vi "Write Toggle enable.vi"(8 "error in (no error)":errorcluster, 10 "Toggle enable":bool, 11 "Motor-Maxon in":refnum<class "Motor-Maxon.lvclass">) -> (0 "error out":errorcluster, 3 "Motor-Maxon out":refnum<class "Motor-Maxon.lvclass">)   [LabVIEW 2013, in "PowderDeposition.lvlib" / "Motor-Maxon.lvclass"]
uses:
  Motor-Maxon.lvclass
  Motor-Maxon.lvclass/Motor-Maxon.ctl
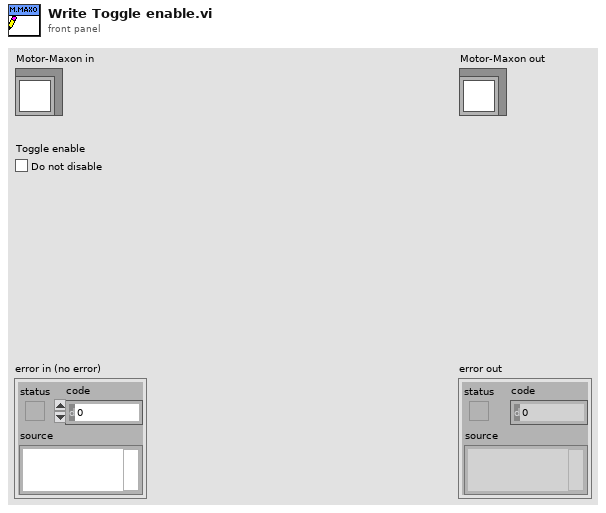
[diagram p1: front panel]
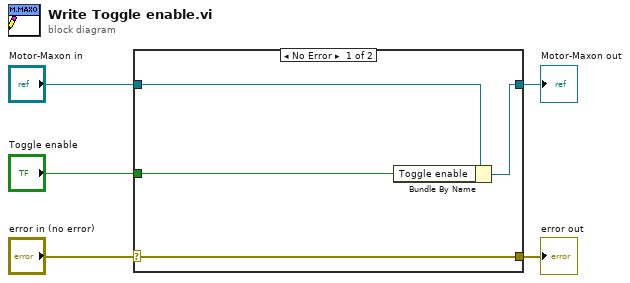
[diagram p0: block diagram]
diagram:
  n1 = case shown="No Error" "error in (no error)" {
    selector: "error in (no error)" -> [w9 w10]
    tunnel: [w9 w10] -> w4
    tunnel: [w7 w11] -> w2
    tunnel: "Motor-Maxon in" -> [w8 w11]
    tunnel: "Toggle enable" -> [w6 _]
    frame No Error {
      n2 = Bundle By Name(cluster=w8, "Toggle enable"=w6) -> (w7:refnum<class "Motor-Maxon.lvclass">)
    }
    frame Error {
    }
  }
  "error out" <- w4
  "Motor-Maxon out" <- w2
